vi "AlliGator Add Phasor Ratio to Plot (with optional dialog).vi"(0 "XYGraph in":refnum<vi>, 5 "Plot ID (-1)":i32=-1, 7 "Phasor Ratio":dbl format="%#.3g", 9 "Time Point":dbl, 11 "error in (no error)":errorcluster, 12 "Interactive?":bool, 13 "New Plot Name":string) -> (3 "Cancelled?":bool, 4 "Sample Abscissa":dbl, 6 "Phasor Ratio":dbl, 10 "# Plots":i32, 14 "Message":string, 15 "error out":errorcluster)   [LabVIEW 2021, in "AlliGator Phasor Ratio.lvlib"]
doc: "Dialog to add individual Phasor Ratio value to a Phasor Ratio plot."
uses:
  AlliGator Phasor Ratio.lvlib
  Graphs/Plot Point Style.ctl
  Graphs/XY Graph/XY Graph Add-Ons.lvlib
  Graphs/Graphs.lvlib
panel:
  in  "Create New Phasor Ratio Plot":bool
  out "Actual Plot ID":i32
  in  "Sample Abscissa":dbl format="%#.3g"
  in  "Cancel Button":bool
  in  "OK Button":bool
  # "Enter sample abscissa for this Phasor Ratio:"
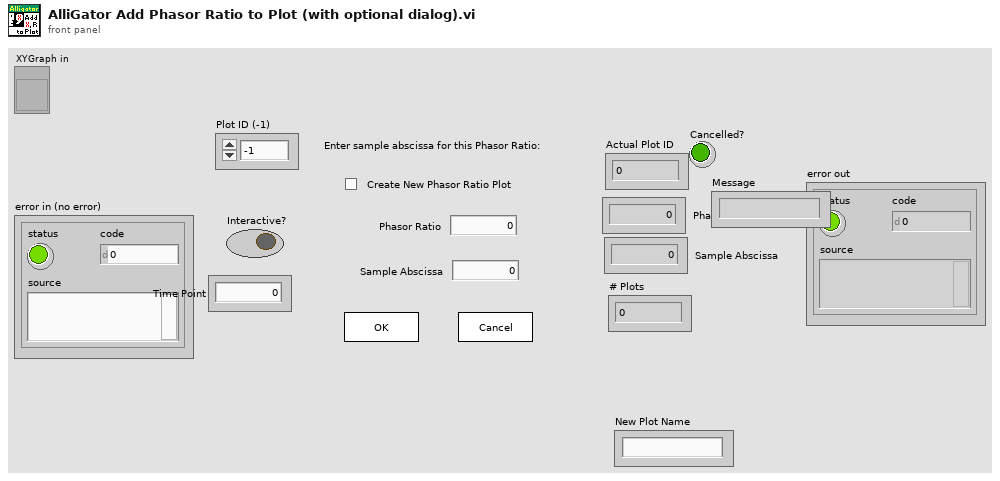
[diagram p1: front panel]
types:
  T1 = enum32{"Invalid", "Standard", "Closed", "Hidden", "Minimized", "Maximized"}
  T2 = typedef "Graphs.lvlib/Plot Point Style.ctl" = enum16{"not defined", "None", "Empty Circle", "Filled Circle", "Thick Circle", "Dotted Circle", "Empty Square", "Filled Square", "Thick Square", "Dotted Square", "Small Filled Square", "Dot", "Cross", "Tiny Cross", "Large X", "Small x", "Diamond", "Small Empty Square"}
  T3 = typedef "XY Graph Add-Ons.lvlib/XY Graph Refnum.ctl" = refnum<vi>
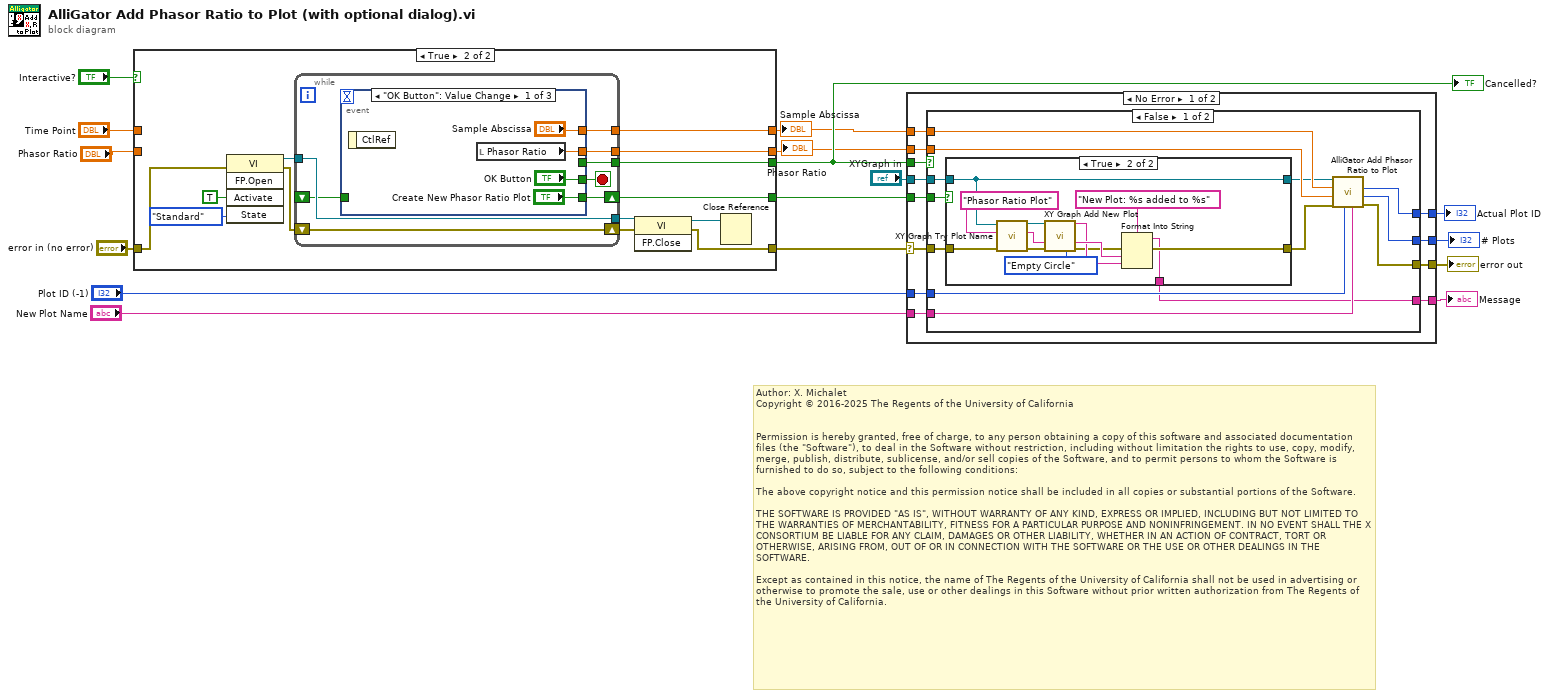
[diagram p0: block diagram]
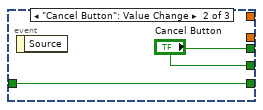
[diagram p6: hidden frame]
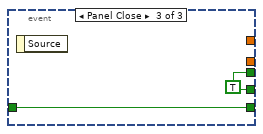
[diagram p7: hidden frame]
diagram:
  # "Author: X. Michalet\nCopyright © 2016-2025 The Regents of the University of California\n \n\nPermission is hereby granted, free of charge, to any person obtaining a copy of this software and associated documentation files (the \"Software\"), to deal in the Software without restriction, including without limitation the rights to use, copy, modify, merge, publish, distribute, sublicense, and/or sell copies of the Software, and to permit persons to whom the Software is furnished to do so, subject to the following conditions:\n\nThe above copyright notice and this permission notice shall be included in all copies or substantial portions of the Software.\n\nTHE SOFTWARE IS PROVIDED \"AS IS\", WITHOUT WARRANTY OF ANY KIND, EXPRESS OR IMPLIED, INCLUDING BUT NOT LIMITED TO THE WARRANTIES OF MERCHANTABILITY, FITNESS FOR A PARTICULAR PURPOSE AND NONINFRINGEMENT. IN NO EVENT SHALL THE X CONSORTIUM BE LIABLE FOR ANY CLAIM, DAMAGES OR OTHER LIABILITY, WHETHER IN AN ACTION OF CONTRACT, TORT OR OTHERWISE, ARISING FROM, OUT OF OR IN CONNECTION WITH THE SOFTWARE OR THE USE OR OTHER DEALINGS IN THE SOFTWARE.\n\nExcept as contained in this notice, the name of The Regents of the University of California shall not be used in advertising or otherwise to promote the sale, use or other dealings in this Software without prior written authorization from The Regents of the University of California."
  n1 = case shown="True" "Interactive?" {
    selector: "Interactive?" -> [w19 _]
    tunnel: "error in (no error)" -> [w18 w28]
    tunnel: [w18 w23] -> w15
    tunnel: [w19 w33] -> w13
    tunnel: [w17 w32] -> w12
    tunnel: [w20 w31] -> w11
    tunnel: "Time Point" -> [w17 _]
    tunnel: "Phasor Ratio" -> [w20 _]
    tunnel: [_ w21] -> w2
    frame False {
    }
    frame True {
      n2 = invoke class="VI" method="FP.Open"(error in=w28, "Activate"=TRUE ("Activate?"), "State"=T1."Standard") -> (reference out=w26:refnum<vi>, error out=w27:errorcluster)  [unwired: 2 in, 3 out]
      n3 = while {
        tunnel: [w40] -> w33
        tunnel: [w38] -> w32
        tunnel: [w37] -> w31
        shift-right: [w39] -> w24
        shift-left: w27 -> [w39]
        tunnel: w26 -> [w36]
        tunnel: [w36] -> w25
        shift-right: [w35] -> w21
        shift-left: _ -> [w34]
        stop <- w41 stop-if-true
        n4 = event shown="[0] \"OK Button\": Value Change" {
          selector: _ -> [_ _ _]
          dyn-events: _ -> [_ _ _]
          timeout: _ -> [_ _ _]
          tunnel: ["OK Button" "Cancel Button" w49] -> w41
          tunnel: [_ "Cancel Button" w49] -> w40
          tunnel: ["Sample Abscissa" _ _] -> w38
          tunnel: [w44 _ _] -> w37
          tunnel: ["Create New Phasor Ratio Plot" w46 w48] -> w35
          tunnel: w34 -> [_ w46 w48]
          event "OK Button": Value Change {
            n5 = event-data() -> ()  [unwired: 1 in, 1 out]
            n6 = local read "Phasor Ratio"() -> (w44:dbl)
          }
          event "Cancel Button": Value Change {
            n7 = event-data() -> ()  [unwired: 1 in, 1 out]
          }
          event Panel Close {
            w49 = TRUE ("Cancel Button")
            n8 = event-data() -> ()  [unwired: 1 in, 1 out]
          }
        }
      }
      n9 = invoke class="VI" method="FP.Close"(reference=w25, error in=w24) -> (reference out=w22:refnum<vi>, error out=w23:errorcluster)  [unwired: 1 in, 1 out]
      n10 = Close Reference(reference=w22) -> ()  [unwired: 1 in, 1 out]
    }
  }
  "Phasor Ratio" <- w11
  "Sample Abscissa" <- w12
  "Cancelled?" <- w13
  n11 = case shown="No Error" w15 {
    selector: w15 -> [w61 w91]
    tunnel: "XYGraph in" -> [w60 _]
    tunnel: w13 -> [w59 _]
    tunnel: w12 -> [w58 _]
    tunnel: w11 -> [w57 _]
    tunnel: [w56 w91] -> w7
    tunnel: "Plot ID (-1)" -> [w55 _]
    tunnel: [w54 _] -> w5
    tunnel: [w53 _] -> w4
    tunnel: "New Plot Name" -> [w52 _]
    tunnel: w2 -> [w51 _]
    tunnel: [w50 _] -> w1
    frame No Error {
      n12 = case shown="False" w59 {
        tunnel: w61 -> [w65 w90]
        tunnel: w60 -> [w66 _]
        tunnel: w57 -> [w73 _]
        tunnel: [w70 w90] -> w56
        tunnel: w58 -> [w74 _]
        tunnel: w55 -> [w71 _]
        tunnel: [w72 _] -> w54
        tunnel: [w69 _] -> w53
        tunnel: w52 -> [w68 _]
        tunnel: w51 -> [w67 _]
        tunnel: [w62 _] -> w50
        frame False {
          n13 = case shown="True" w67 {
            tunnel: w66 -> [w75 w81]
            tunnel: w65 -> [w76 w83]
            tunnel: [w76 w79] -> w64
            tunnel: [w75 w81] -> w63
            tunnel: [_ w77] -> w62
            frame False {
            }
            frame True {
              n14 = call "XY Graph Try Plot Name.vi"("Error In"=w83, "Plot Name in"="Phasor Ratio Plot", "XY Graph Refnum"=w81) -> ("Error Out"=w82:errorcluster, "Plot Name out"=w86:string, "XY Graph Refnum"=w87:T3)  [unwired: 5 in, 1 out]
              n15 = call "XY Graph Add New Plot.vi"("Multiplot XY Graph"=w87, "New Plot Name in"=w86, "error in (no error)"=w82, "Point Style (Dot)"=Plot_Point_Style."Empty Circle") -> ("XY Graph Caption"=w88:string, "New Plot Name out"=w89:string, "error out"=w85:errorcluster)  [unwired: 8 in, 1 out]
              n16 = Format Into String(format string="New Plot: %s added to %s", error in=w85, w89, w88) -> (resulting string=w77:string, error out=w79:errorcluster)  [unwired: 1 in]
            }
          }
          n17 = call "AlliGator Add Phasor Ratio to Plot.vi"("New Plot Name"=w68, "Plot ID (-1)"=w71, "error in (no error)"=w64, "Phasor Ratio"=w73, "Abscissa"=w74, "Phasor Ratio Graph refnum"=w63) -> ("error out"=w70:errorcluster, "# Plots"=w72:i32, "Actual Plot ID"=w69:i32)  [unwired: 2 in, 1 out]
        }
        frame True {
        }
      }
    }
    frame Error {
    }
  }
  "error out" <- w7
  "# Plots" <- w5
  "Actual Plot ID" <- w4
  "Message" <- w1
